vi "color 1.vi"(7 "ROI Descriptor":T1 {"Contours"."Type" items=["No Selection", "Point", "Line", "Rectangle", "Oval", "Polygon", "Free", "Annulus", "Unused2", "Unused3", "Broken Line", "Free Hand Line", "Rotated Rectangle"]}, 8 "error in (no error)":errorcluster, 10 "Image 2":T2, 11 "color":path) -> (2 "Image":T2(plugin-control), 3 "Class":string)   [LabVIEW 2015]
uses:
  <vilib>/vision/Image Controls.llb/IMAQ Image.ctl
  <vilib>/vision/NI_Vision_Development_Module.lvlib
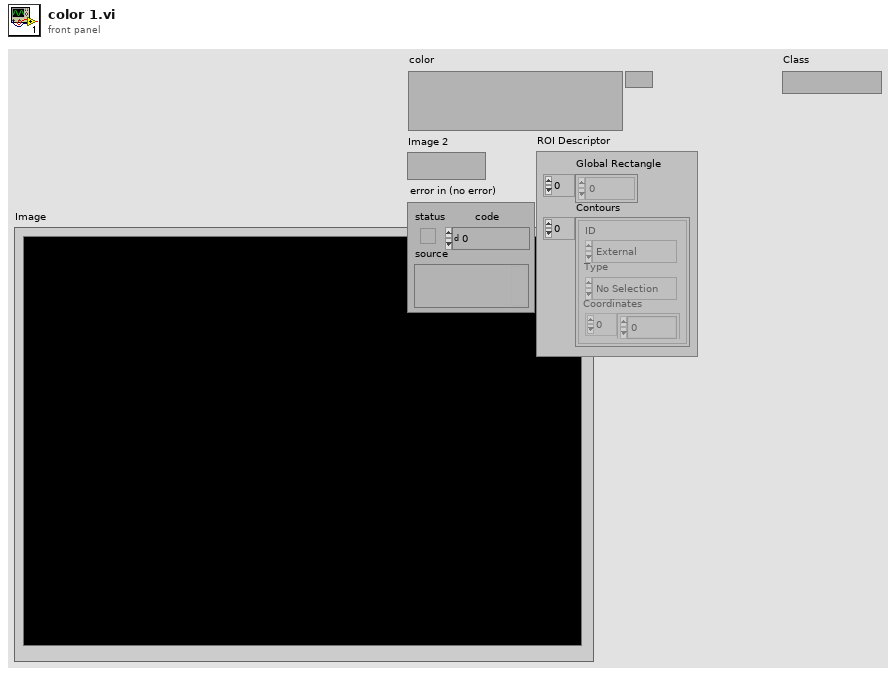
[diagram p1: front panel]
types:
  T1 = cluster{"Global Rectangle":i32[], "Contours":cluster{"ID":enum32{"External", "Internal"}, "Type":u32, "Coordinates":i32[]}[]}
  T2 = typedef "IMAQ Image.ctl" = refnum<image>
  T3 = typedef "IMAQ Classifier Session.ctl" = refnum<k1>
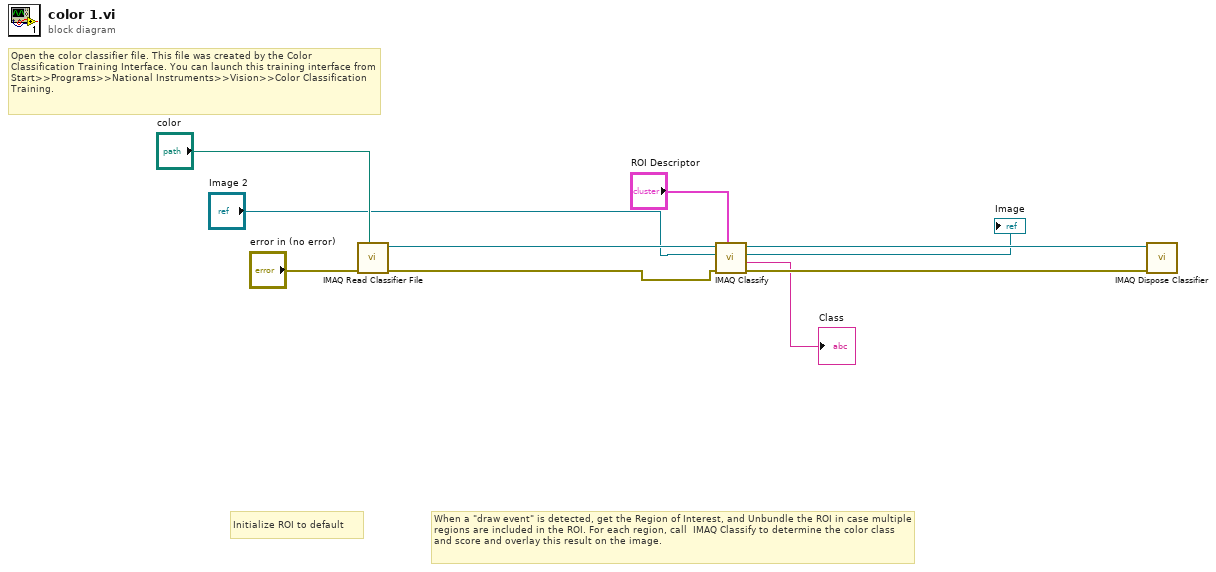
[diagram p0: block diagram]
diagram:
  # "Open the color classifier file. This file was created by the Color Classification Training Interface. You can launch this training interface from Start>>Programs>>National Instruments>>Vision>>Color Classification Training."
  # "Initialize ROI to default"
  # "When a \"draw event\" is detected, get the Region of Interest, and Unbundle the ROI in case multiple regions are included in the ROI. For each region, call  IMAQ Classify to determine the color class and score and overlay this result on the image."
  n1 = call "IMAQ Read Classifier File"("File Path"="color", "error in (no error)"="error in (no error)") -> ("error out"=w1:errorcluster, "Classifier Session"=w10:T3)  [unwired: 2 in, 6 out]
  n2 = call "IMAQ Classify"("ROI Descriptor"="ROI Descriptor", "error in (no error)"=w1, "Image"="Image 2", "Classifier Session"=w10) -> ("error out"=w5:errorcluster, "Class"=→"Class":string, "Image (dup)"=→"Image":T2, "Classifier Session (dup)"=w6:T3)  [unwired: 4 out]
  n3 = call "IMAQ Dispose Classifier"("error in (no error)"=w5, "Classifier Session"=w6) -> ()  [unwired: 10 out]
